vi "CaseParams.vi"(8 "avg num":sgl format="%.2f", 10 "Number of Scans":i32, 11 "File Name In":string) -> (3 "Scan Params":T1 {"Digitizer delay\n (ms)" format="%.2f"; "avg num" format="%.2f"})   [LabVIEW 2022 SP3]
uses:
  ScanningControl/Motion Controllers/-MotionRoutines/MotionGlobals.vi
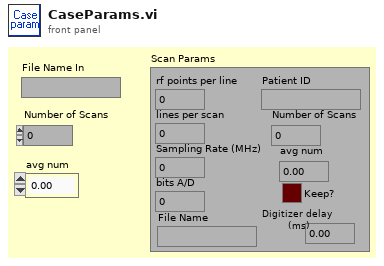
[diagram p1: front panel]
types:
  T1 = cluster{"rf points per line":u16, "lines per scan":u16, "Sampling Rate (MHz)":i32, "bits A/D":i32, "File Name":string, "Patient ID":string, "Number of Scans":i32, "avg num":dbl, "Keep?":bool, "Digitizer delay\n (ms) ":dbl}
  T2 = cluster{"rf points per line":void, i32, "Sampling Rate (MHz)":dbl, "bits A/D":void, "File Name In":string, "Patient ID":void, "Number of Scans":i32, "avg num":sgl, "Save?":bool, i32}
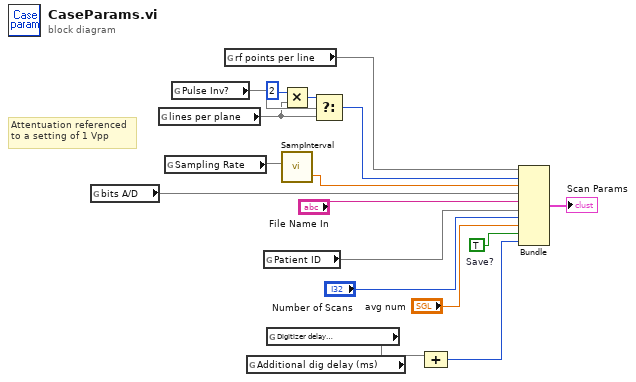
[diagram p0: block diagram]
diagram:
  w13 = TRUE  # Save?
  # "Attentuation referenced\nto a setting of 1 Vpp"
  n1 = global read "MotionGlobals.vi" "bits A/D"() -> (w3)
  n2 = global read "MotionGlobals.vi" "lines per plane"() -> (w5)
  n3 = global read "MotionGlobals.vi" "Sampling Rate"() -> (w17)
  n4 = global read "MotionGlobals.vi" "Pulse Inv?"() -> (w6)
  n5 = global read "MotionGlobals.vi" "rf points per line"() -> (w16)
  n6 = global read "MotionGlobals.vi" "Additional dig delay (ms)"() -> (w11)
  n7 = global read "MotionGlobals.vi" "Patient ID"() -> (w15)
  n8 = global read "MotionGlobals.vi" "Digitizer delay\n (ms)"() -> (w12)
  n9 = Multiply(x=2, y=w5) -> (x*y=w4:i32)
  n10 = call "SampInterval.vi"("Sampling Rate"=w17) -> ("Sampling Rate (MHz)"=w18:dbl)  [unwired: 2 out]
  n11 = Select(t=w4, s=w6, f=w5) -> (s? t:f=w7:i32)
  n12 = Compound Arithmetic op=ADD(w12, w11) -> (w10:i32)
  n13 = Bundle("rf points per line"=w16, w7, "Sampling Rate (MHz)"=w18, "bits A/D"=w3, "File Name In"="File Name In", "Patient ID"=w15, "Number of Scans"="Number of Scans", "avg num"="avg num", "Save?"=w13, w10) -> (→"Scan Params":T2)  [unwired: 1 out]
